vi "Save Confluence Connection Settings.vi"(8 "Error in":errorcluster caption="Error in (no error)", 10 "Confluence Connection Settings":T1, 11 "Settings Path":path) -> (0 "Error out":errorcluster)   [LabVIEW 2023, in "VIDoc Printer - Confluence.lvlib" / "VIDoc Settings - Confluence.lvclass"]
uses:
  VIDoc Settings - Confluence.lvclass
  f2867cc3-0f83-4cb6-a4b6-5f1cf02df459.vi
  VIDoc Settings/VIDoc Settings.lvclass
  Confluence Connection Settings.ctl
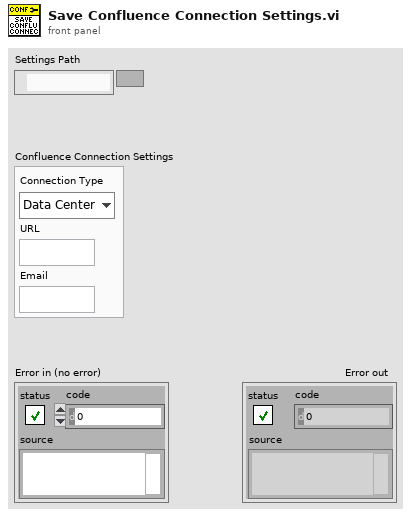
[diagram p1: front panel]
types:
  T1 = typedef "VIDoc Printer - Confluence.lvlib/VIDoc Settings - Confluence.lvclass/Confluence Connection Settings.ctl" = cluster{"Connection Type":enum16{"Data Center", "Cloud"}, "URL":string, "Email":string}
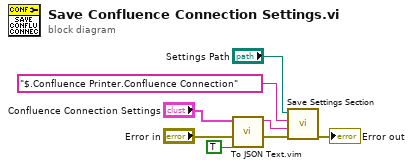
[diagram p0: block diagram]
diagram:
  n1 = call "To JSON Text.vim"("Pretty Print?"=TRUE, "error in (no error)"="Error in", "Anything"="Confluence Connection Settings") -> ("error out"=w7:errorcluster, "<JSON>"=w5:string)  [unwired: 7 in]
  n2 = call "Save Settings Section.vi"("Error in"=w7, "JSON Object"=w5, "Section Name"="$.Confluence Printer.Confluence Connection", "JSON Settings Path"="Settings Path") -> ("Error out"=→"Error out":errorcluster)  [unwired: 7 in]
